vi "write state.vi"(8 "error in (no error)":errorcluster, 10 "State":string, 11 "FWCS_ACS_Iterator in":refnum<class "FWCS_ACS_Iterator.lvclass">) -> (0 "error out":errorcluster, 3 "FWCS_ACS_Iterator out":refnum<class "FWCS_ACS_Iterator.lvclass">)   [LabVIEW 2018, in "FWCS_ACS_Iterator.lvclass"]
uses:
  FWCS_ACS_Iterator.lvclass
  FWCS_ACS_Iterator.lvclass/FWCS_ACS_Iterator.ctl
  State Machine/State Machine.lvclass
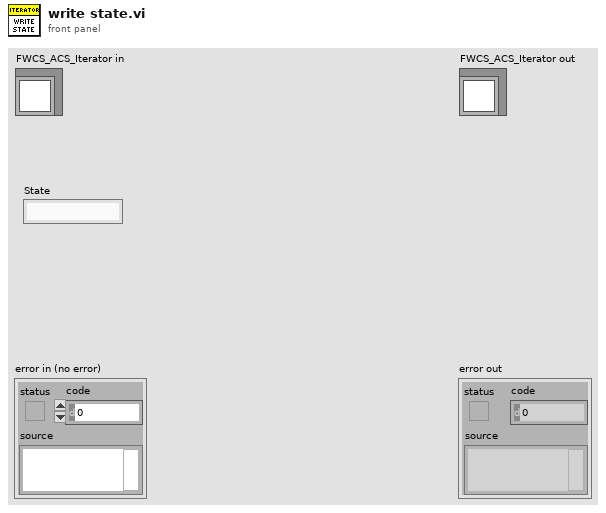
[diagram p1: front panel]
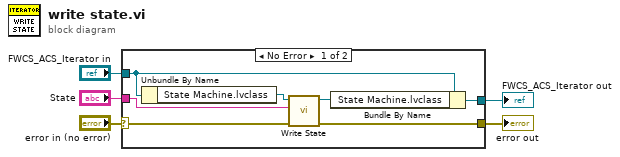
[diagram p0: block diagram]
diagram:
  n1 = case shown="No Error" "error in (no error)" {
    selector: "error in (no error)" -> [w8 w14]
    tunnel: [w7 w14] -> w4
    tunnel: [w11 w13] -> w2
    tunnel: "FWCS_ACS_Iterator in" -> [w12 w13]
    tunnel: "State" -> [w6 _]
    frame No Error {
      n2 = Unbundle By Name(w12) -> ("State Machine.lvclass"=w10:refnum<class "State Machine.lvclass">)
      n3 = call-dynamic "Write State.vi"("error in (no error)"=w8, "State"=w6, "State Machine in"=w10) -> ("error out"=w7:errorcluster, "State Machine out"=w9:refnum<class "State Machine.lvclass">)  [unwired: 7 in]
      n4 = Bundle By Name(cluster=w12, "State Machine.lvclass"=w9) -> (w11:refnum<class "FWCS_ACS_Iterator.lvclass">)
    }
    frame Error {
    }
  }
  "error out" <- w4
  "FWCS_ACS_Iterator out" <- w2
